vi "broadfit.vi"(0 "input":dbl[][](array[numeric]) format="%.5f", 1 "T mean start":dbl=2.35 format="%.2f", 2 "fit cycles":u32=50, 3 "n norm":u8=7, 5 "T min":dbl format="%.2f", 7 "T max":dbl=20.0 format="%.2f", 9 "# points":dbl=1023.0 format="%.2f", 11 "R_offset start":dbl format="%.2f", 12 "Delta T start":dbl=1.15 format="%.2f", 13 "adjustment":dbl=1.0 format="%.3f") -> (4 "T mean final":dbl=2.35 format="%.2f", 6 "Delta T final":dbl=1.15 format="%.2f", 8 "R_offset final":dbl format="%.2f", 10 "r_0":dbl format="%.2f", 15 "sumsqu":dbl format="%.6f")   [LabVIEW 2018]
panel:
  out "running adj.":dbl format="%.3f"
  out "count":u32
  out "R_offset running":dbl format="%.2f"
  out "Delta T running":dbl=1.15 format="%.2f"
  out "T mean running":dbl=2.35 format="%.2f"
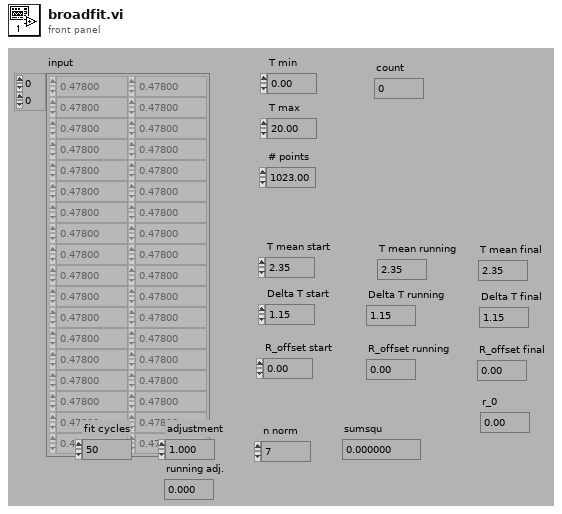
[diagram p1: front panel]
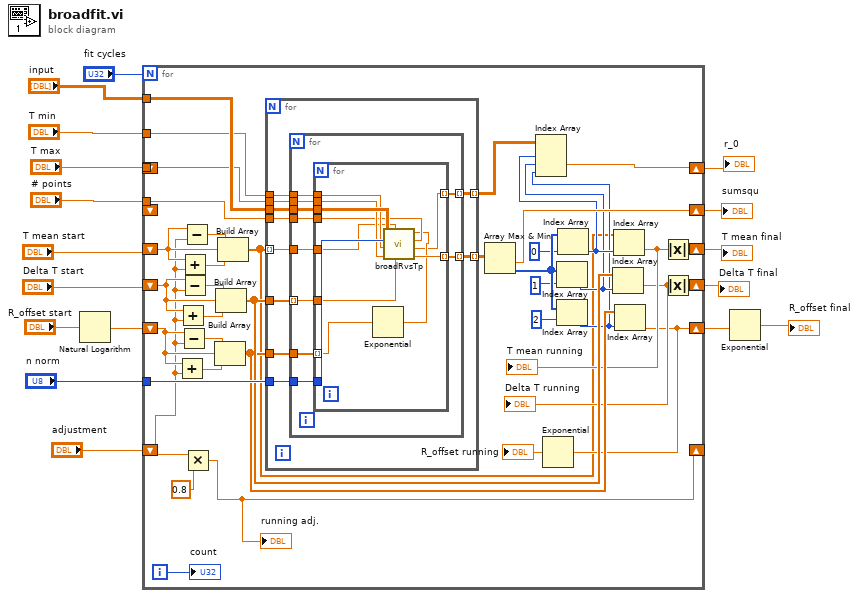
[diagram p0: block diagram]
diagram:
  n1 = Natural Logarithm(1:"R_offset start") -> (0:w7:dbl)
  n2 = for {
    N: "fit cycles" -> [_]
    tunnel: "input" -> [w46]
    tunnel: "T min" -> [w44]
    tunnel: "T max" -> [w43]
    tunnel: "# points" -> [w42]
    shift-right: [w19] -> w6
    shift-left: "T mean start" -> [w54]
    shift-right: [w18] -> w5
    shift-left: "Delta T start" -> [w48]
    shift-right: [w32] -> w4
    shift-left: w7 -> [w47]
    tunnel: "n norm" -> [w45]
    shift-right: [w28] -> _
    shift-left: "adjustment" -> [w30]
    shift-right: [w26] -> w2
    shift-left: _ -> [_]
    shift-right: [w21] -> w1
    shift-left: _ -> [_]
    i -> [w31]
    n3 = Add(x=w47, y=w30) -> (x+y=w49:dbl)
    n4 = Add(x=w48, y=w30) -> (x+y=w51:dbl)
    n5 = Subtract(x=w47, y=w30) -> (x-y=w50:dbl)
    n6 = Add(x=w54, y=w30) -> (x+y=w53:dbl)
    n7 = Subtract(x=w48, y=w30) -> (x-y=w52:dbl)
    n8 = Subtract(x=w54, y=w30) -> (x-y=w55:dbl)
    n9 = Multiply(x=w30, y=0.8) -> (x*y=w28:dbl)
    "running adj." <- w28
    n10 = Build Array(w50, w47, w49) -> (w35:dbl[])
    n11 = Build Array(w52, w48, w51) -> (w36:dbl[])
    n12 = Build Array(w55, w54, w53) -> (w20:dbl[])
    n13 = for {
      tunnel: w20 -> [w65] mode=indexing
      tunnel: w36 -> [w64]
      tunnel: w35 -> [w63]
      tunnel: w46 -> [w62]
      tunnel: w45 -> [w61]
      tunnel: w44 -> [w60]
      tunnel: w43 -> [w59]
      tunnel: w42 -> [w58]
      tunnel: [w57] -> w41 mode=indexing
      tunnel: [w56] -> w23 mode=indexing
      n14 = for {
        tunnel: w65 -> [w75]
        tunnel: w64 -> [w74] mode=indexing
        tunnel: w63 -> [w73]
        tunnel: w62 -> [w72]
        tunnel: w61 -> [w71]
        tunnel: w60 -> [w70]
        tunnel: w59 -> [w69]
        tunnel: w58 -> [w68]
        tunnel: [w67] -> w57 mode=indexing
        tunnel: [w66] -> w56 mode=indexing
        n15 = for {
          tunnel: w75 -> [w81]
          tunnel: w74 -> [w80]
          tunnel: w73 -> [w79] mode=indexing
          tunnel: w72 -> [w86]
          tunnel: w71 -> [w85]
          tunnel: w70 -> [w84]
          tunnel: w69 -> [w83]
          tunnel: w68 -> [w82]
          tunnel: [w78] -> w67 mode=indexing
          tunnel: [w76] -> w66 mode=indexing
          n16 = Exponential(1:w79) -> (0:w77:dbl)
          n17 = call "broadRvsTp.vi"("# points"=w82, "R_offset"=w77, "Delta T"=w80, "T mean"=w81, "T max"=w83, "T min"=w84, "n norm?"=w85, 9:w86) -> ("sumsqu"=w78:dbl, "r_0"=w76:dbl)
        }
      }
    }
    n18 = Array Max & Min(array=w41) -> (min value=w26:dbl, min index (indices)=w40:i32[])  [unwired: 2 out]
    n19 = Index Array(array=w40, index=1) -> (element=w24:i32)
    n20 = Index Array(array=w40, index=2) -> (element=w22:i32)
    n21 = Index Array(array=w40, index=0) -> (element=w25:i32)
    n22 = Index Array(array=w23, index (dim 0)=w25, index (dim 1)=w24, index (dim 2)=w22) -> (element=w21:dbl)
    n23 = Index Array(array=w36, index=w24) -> (element=w33:dbl)
    "Delta T running" <- w33
    n24 = Index Array(array=w20, index=w25) -> (element=w34:dbl)
    "T mean running" <- w34
    n25 = Index Array(array=w35, index=w22) -> (element=w32:dbl)
    n26 = Exponential(1:w32) -> (0:→"R_offset running":dbl)
    n27 = Absolute Value(x=w34) -> (abs(x)=w19:dbl)
    n28 = Absolute Value(x=w33) -> (abs(x)=w18:dbl)
    "count" <- w31
  }
  "T mean final" <- w6
  "Delta T final" <- w5
  "sumsqu" <- w2
  "r_0" <- w1
  n29 = Exponential(1:w4) -> (0:→"R_offset final":dbl)
